vi "HFR500 Set Range.vi"(0 "Ch number":i32=1 min=1 max=4, 1 "ppm Range":T1) -> (2 "Correctly Set?":bool, 3 "Returned Range Code":string, 4 "error out":errorcluster)   [LabVIEW 2020]
uses:
  HFR500 ppm Range.ctl
panel:
  out "Check Response":string
  out "TX String (ASCII) 2":string
  out "TCP Connected":bool
  out "RX String (ASCII)":string
  out "TX String (ASCII)":string
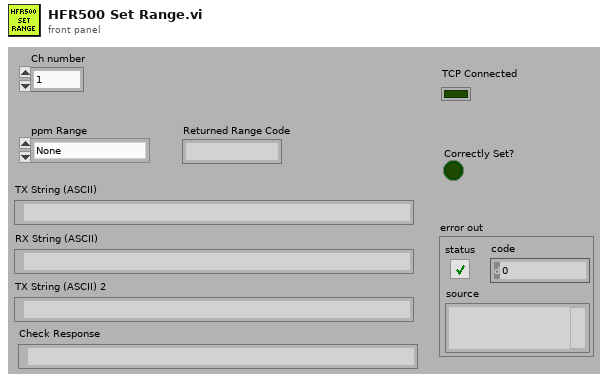
[diagram p1: front panel]
types:
  T1 = typedef "HFR500 ppm Range.ctl" = enum16{"None", "1,000", "2,000", "5,000", "10,000", "20,000", "50,000", "100,000", "200,000"}
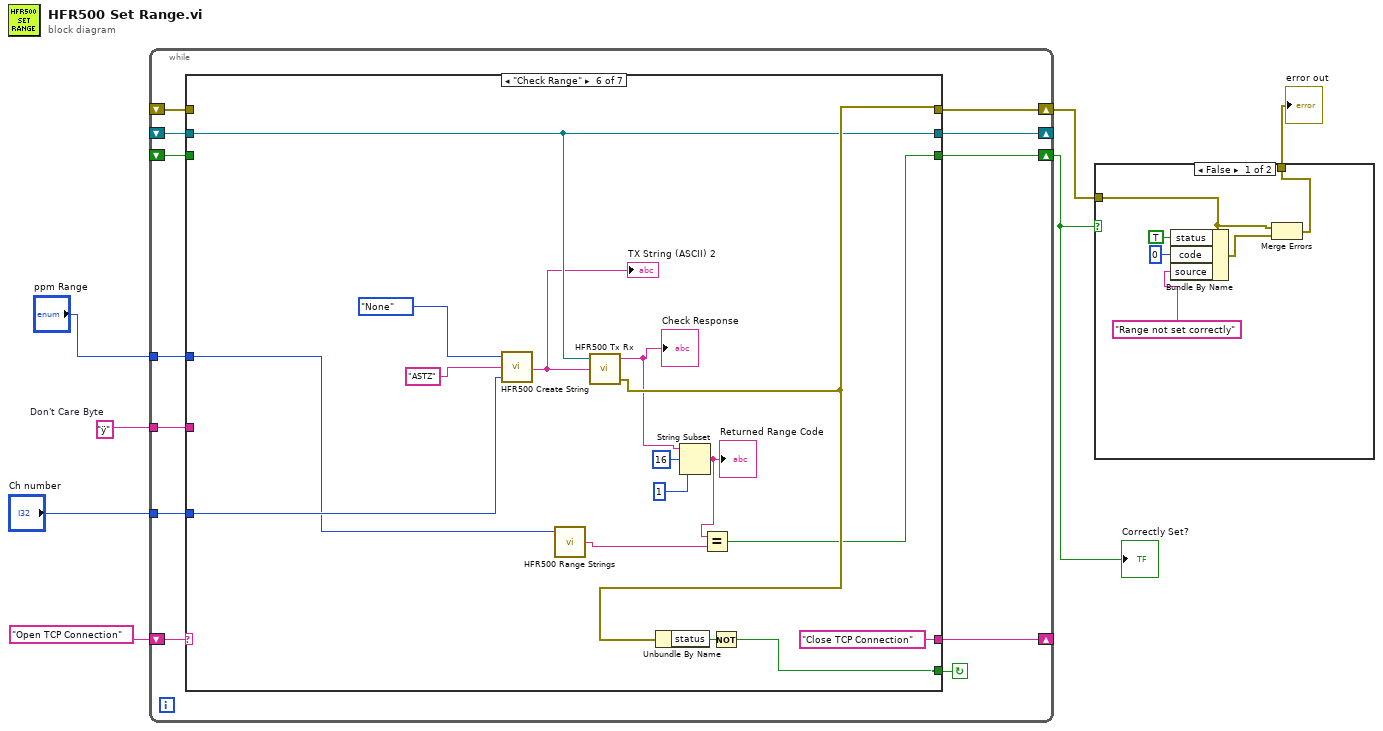
[diagram p0: block diagram]
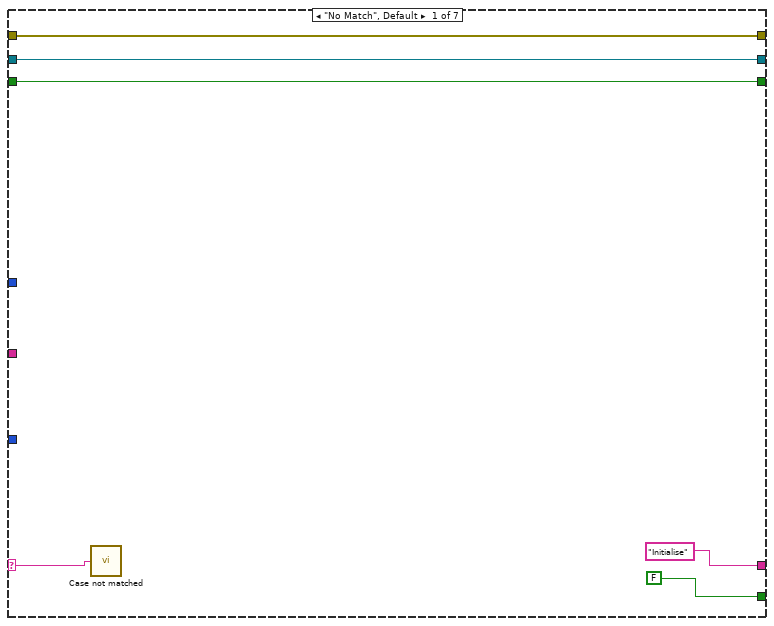
[diagram p3: hidden frame]
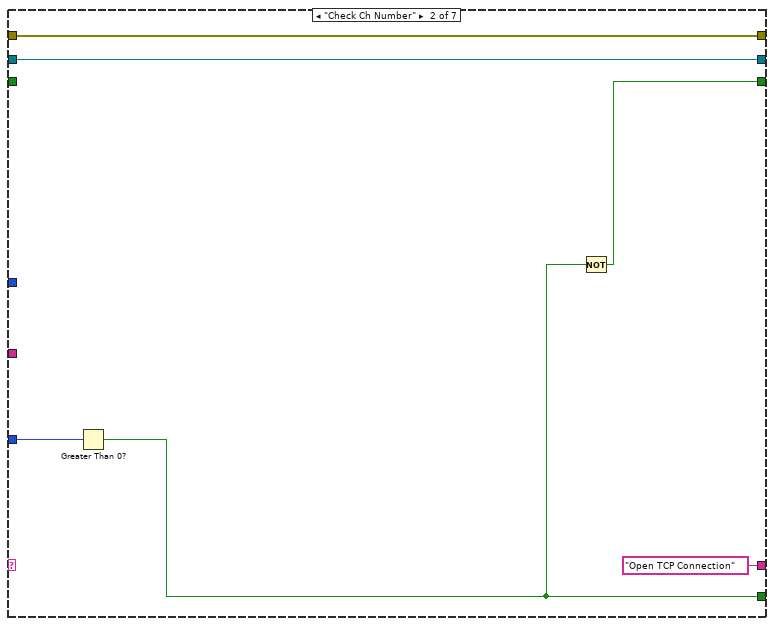
[diagram p4: hidden frame]
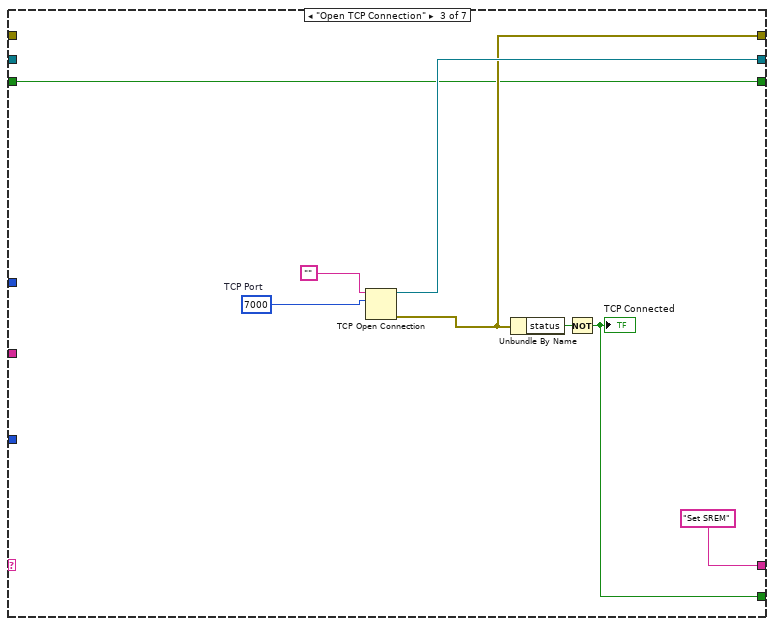
[diagram p5: hidden frame]
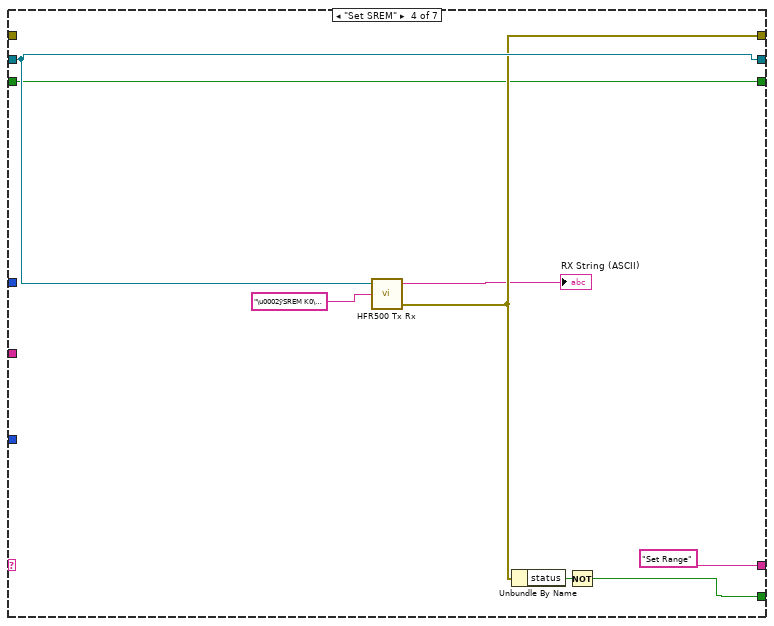
[diagram p6: hidden frame]
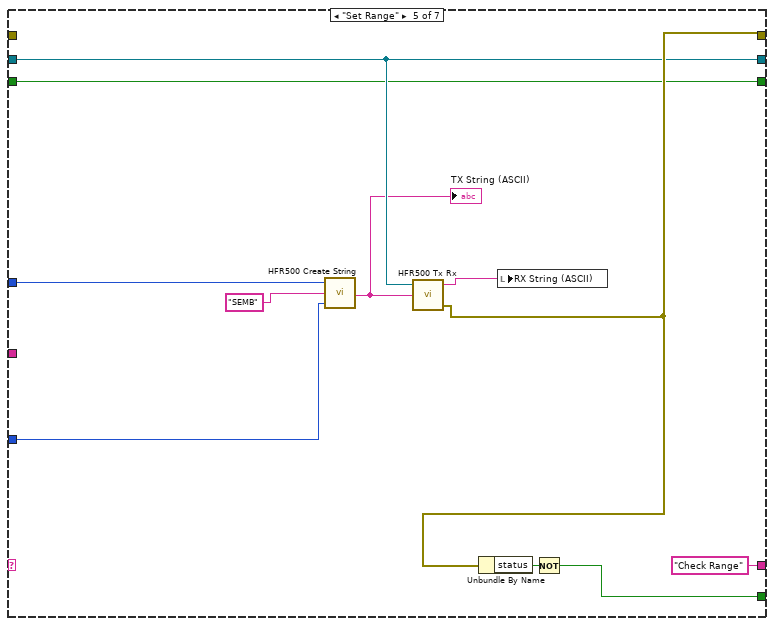
[diagram p7: hidden frame]
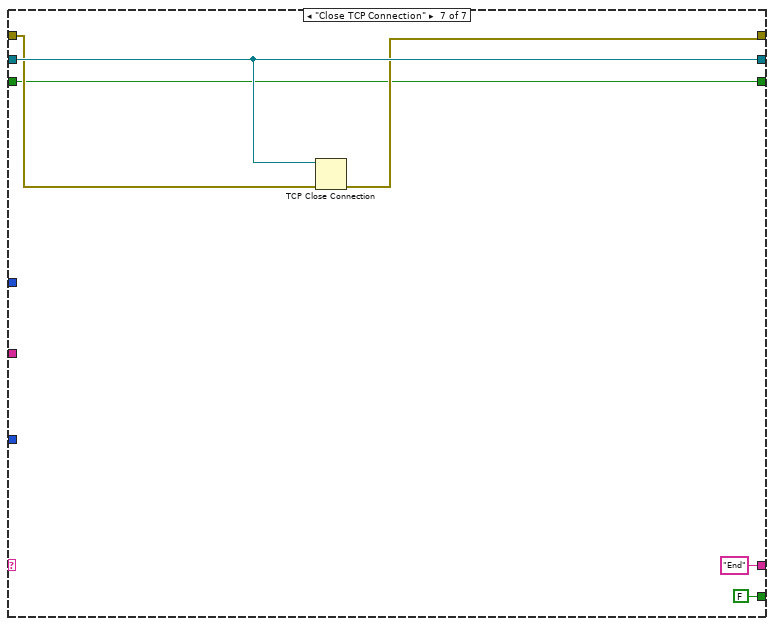
[diagram p8: hidden frame]
diagram:
  w6 = "ÿ"  # Don't Care Byte
  n1 = while {
    shift-left: "Open TCP Connection" -> [w17]
    shift-right: [w18] -> _
    shift-right: [w16] -> _
    shift-left: _ -> [w13]
    shift-right: [w15] -> w1
    shift-left: _ -> [w14]
    tunnel: w6 -> [w12]
    tunnel: "Ch number" -> [w11]
    tunnel: "ppm Range" -> [w10]
    shift-right: [w8] -> w3
    shift-left: _ -> [w9]
    stop <- w19 continue-if-true
    n2 = case shown="\"Check Range\"" w17 {
      selector: w17 -> [w23 _ _ _ _ _ _]
      tunnel: [FALSE w27 w35 w43 w57 w73 FALSE] -> w19
      tunnel: ["Initialise" "Open TCP Connection" "Set SREM" "Set Range" "Check Range" "Close TCP Connection" "End"] -> w18
      tunnel: [w21 w30 w37 w46 w53 w70 w80] -> w16
      tunnel: [w22 w31 w36 w44 w54 w71 w78] -> w15
      tunnel: w14 -> [w22 w31 _ _ _ _ w79]
      tunnel: w13 -> [w21 w30 _ w46 w53 w70 w80]
      tunnel: w12 -> [_ _ _ _ _ _ _]
      tunnel: w11 -> [_ w28 _ _ w50 w67 _]
      tunnel: w10 -> [_ _ _ _ w49 w62 _]
      tunnel: w9 -> [w20 _ w32 w40 w48 _ w75]
      tunnel: [w20 w26 w32 w40 w48 w59 w75] -> w8
      frame "No Match", Default {
        n3 = call "Case not matched.vi"("Case Name not Matched"=w23) -> ()
      }
      frame "Check Ch Number" {
        n4 = Greater Than 0?(x=w28) -> (x > 0?=w27:bool)
        n5 = Not(x=w27) -> (.not. x?=w26:bool)
      }
      frame "Open TCP Connection" {
        w33 = u16 7000  # TCP Port
        n6 = TCP Open Connection(address="", remote port or service name=w33) -> (connection ID=w37:refnum<k5>, error out=w36:errorcluster)  [unwired: 3 in]
        n7 = Unbundle By Name(w36) -> ("status"=w38:bool)
        n8 = Not(x=w38) -> (.not. x?=w35:bool)
        "TCP Connected" <- w35
      }
      frame "Set SREM" {
        n9 = call "HFR500 Tx Rx.vi"("String to Write"="\u0002ÿSREM K0\u0003" ("Initial string"), "TCP Network Connection in"=w46) -> ("error out"=w44:errorcluster, "RX String (ASCII)"=→"RX String (ASCII)":string)  [unwired: 2 in]
        n10 = Unbundle By Name(w44) -> ("status"=w45:bool)
        n11 = Not(x=w45) -> (.not. x?=w43:bool)
      }
      frame "Set Range" {
        n12 = call "HFR500 Create String.vi"("Ch number"=w50, "Command"="SEMB", "ppm Range"=w49) -> ("TX String (ASCII)"=w51:string)  [unwired: 1 in, 1 out]
        "TX String (ASCII)" <- w51
        n13 = call "HFR500 Tx Rx.vi"("String to Write"=w51, "TCP Network Connection in"=w53) -> ("error out"=w54:errorcluster, "RX String (ASCII)"=w55:string)  [unwired: 2 in]
        n14 = Unbundle By Name(w54) -> ("status"=w58:bool)
        n15 = local write "RX String (ASCII)"(w55) -> ()
        n16 = Not(x=w58) -> (.not. x?=w57:bool)
      }
      frame "Check Range" {
        n17 = call "HFR500 Create String.vi"("Ch number"=w67, "Command"="ASTZ", "ppm Range"=HFR500_ppm_Range."None") -> ("TX String (ASCII)"=w68:string)  [unwired: 1 in, 1 out]
        "TX String (ASCII) 2" <- w68
        n18 = call "HFR500 Range Strings.vi"("ppm Range"=w62) -> ("Range Digit"=w61:string)  [unwired: 3 in, 1 out]
        n19 = call "HFR500 Tx Rx.vi"("String to Write"=w68, "TCP Network Connection in"=w70) -> ("error out"=w71:errorcluster, "RX String (ASCII)"=w63:string)  [unwired: 2 in]
        "Check Response" <- w63
        n20 = Unbundle By Name(w71) -> ("status"=w74:bool)
        n21 = String Subset(string=w63, offset (0)=16, length (rest)=1 ("length (rest)")) -> (substring=w60:string)
        "Returned Range Code" <- w60
        n22 = Equal?(x=w60, y=w61) -> (x = y?=w59:bool)
        n23 = Not(x=w74) -> (.not. x?=w73:bool)
      }
      frame "Close TCP Connection" {
        n24 = TCP Close Connection(connection ID=w80, error in (no error)=w79) -> (error out=w78:errorcluster)  [unwired: 1 in, 1 out]
      }
    }
  }
  "Correctly Set?" <- w3
  n25 = case shown="False" w3 {
    tunnel: [w82 w87] -> w2
    tunnel: w1 -> [w83 w87]
    frame False {
      n26 = Bundle By Name(cluster=w83, "status"=TRUE, "code"=0, "source"="Range not set correctly") -> (w84:errorcluster)
      n27 = Merge Errors(w83, w84) -> (w82:errorcluster)
    }
    frame True {
    }
  }
  "error out" <- w2
